vi "Defer Updates.vi"(8 "Error In":errorcluster, 10 "Defer Panel Updates":bool=TRUE, 11 "Cluster":T1) -> (0 "Error Out":errorcluster, 3 "Cluster Out":T1)   [LabVIEW 2019, in "LSS.lvlib"]
doc: "Simple VI used to defer panel updates before multiple UI changes are made."
uses:
  LSS.lvlib
  Before UI References.ctl
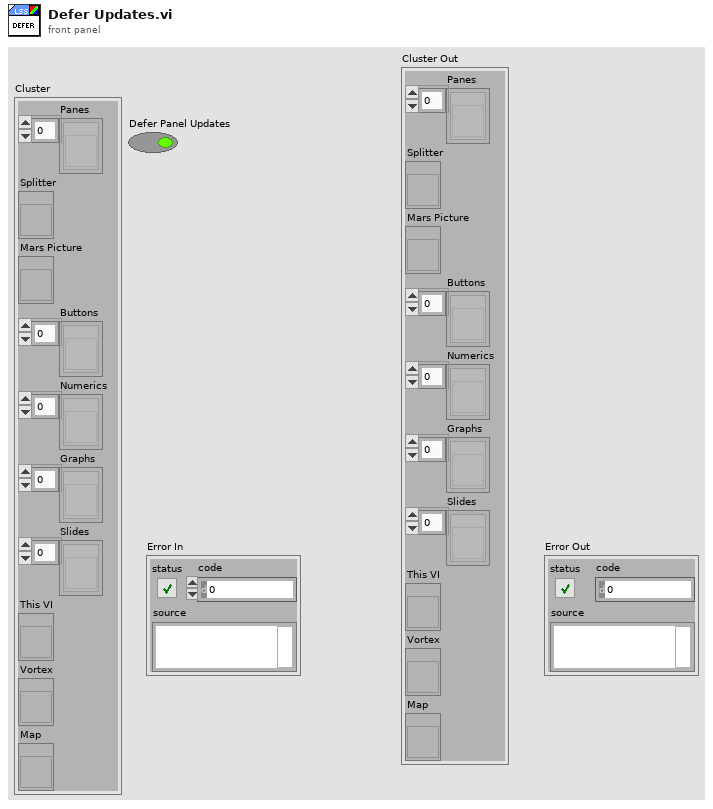
[diagram p1: front panel]
types:
  T1 = typedef "LSS.lvlib/Before UI References.ctl" = cluster{"Panes":refnum<vi>[], "Splitter":refnum<vi>, "Mars Picture":refnum<vi>, "Buttons":refnum<vi>[], "Numerics":refnum<vi>[], "Graphs":refnum<vi>[], "Slides":refnum<vi>[], "This VI":refnum<vi>, "Vortex":refnum<vi>, "Map":refnum<vi>}
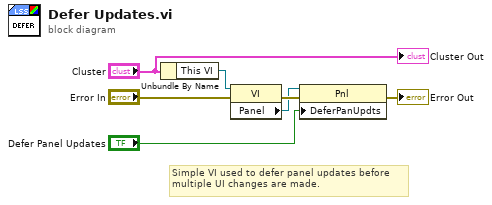
[diagram p0: block diagram]
diagram:
  # "Simple VI used to defer panel updates before\nmultiple UI changes are made."
  n1 = Unbundle By Name("Cluster") -> ("This VI"=w3:refnum<vi>)
  n2 = property class="VI"(reference=w3, error in="Error In") -> (error out=w6:errorcluster, "Panel"=w4:refnum<vi>)  [unwired: 1 out]
  n3 = property class="Pnl"(reference=w4, error in=w6, "DeferPanUpdts"="Defer Panel Updates") -> (error out=→"Error Out":errorcluster)  [unwired: 1 out]
  "Cluster Out" <- "Cluster"
